vi "STM Read Message (Serial).vi"(6 "Options":T2={"Ignore Timeout Error"=TRUE, "timeout ms (1000)"=1000}, 8 "error in":errorcluster, 11 "Connection Info":T4) -> (0 "error out":errorcluster, 1 "Name":T3, 2 "data string":string, 3 "Connection Info Out":T4, 4 "Data Info":T1, 5 "Timed Out?":bool)   [LabVIEW 2014, in "QwaveSys Raspberry Pi Library.lvlib"]
doc: "This VI reads an incoming package of data from a host. This VI parses the package and extracts the data name and type as described in the meta data.\n\nFor the package to be parsed correctly, the meta data must be consistent in both the sender and the receiver. The data is packaged based on the existing meta data on the sender. \n\nUse the \"STM Read Meta Data\" and \"STM Write Meta Data\" VIs to ensure that both client and server have the same meta data.\n\nThe data is returned as a string. It is the responsibility of the user to cast it to the appropriate type."
uses:
  QwaveSys Raspberry Pi Library.lvlib
  stm_Serial Connection Info.ctl
  _SubVIs/stm_MetaDataElement.ctl
  stm_Serial Read Options.ctl
  stm_Serial Data Info.ctl
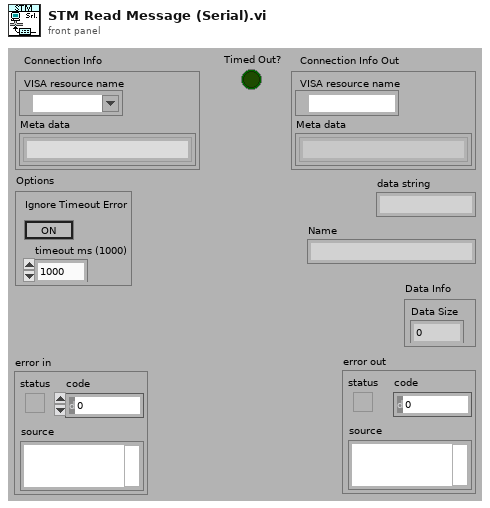
[diagram p1: front panel]
types:
  T1 = typedef "QwaveSys Raspberry Pi Library.lvlib/stm_Serial Data Info.ctl" = cluster{"Data Size":u32}
  T2 = typedef "QwaveSys Raspberry Pi Library.lvlib/stm_Serial Read Options.ctl" = cluster{"Ignore Timeout Error":bool, "timeout ms (1000)":u32}
  T3 = typedef "QwaveSys Raspberry Pi Library.lvlib/stm_MetaDataElement.ctl" = string
  T4 = typedef "QwaveSys Raspberry Pi Library.lvlib/stm_Serial Connection Info.ctl" = cluster{"VISA resource name":refnum<visa-resource-name>, "Meta data":T3[]}
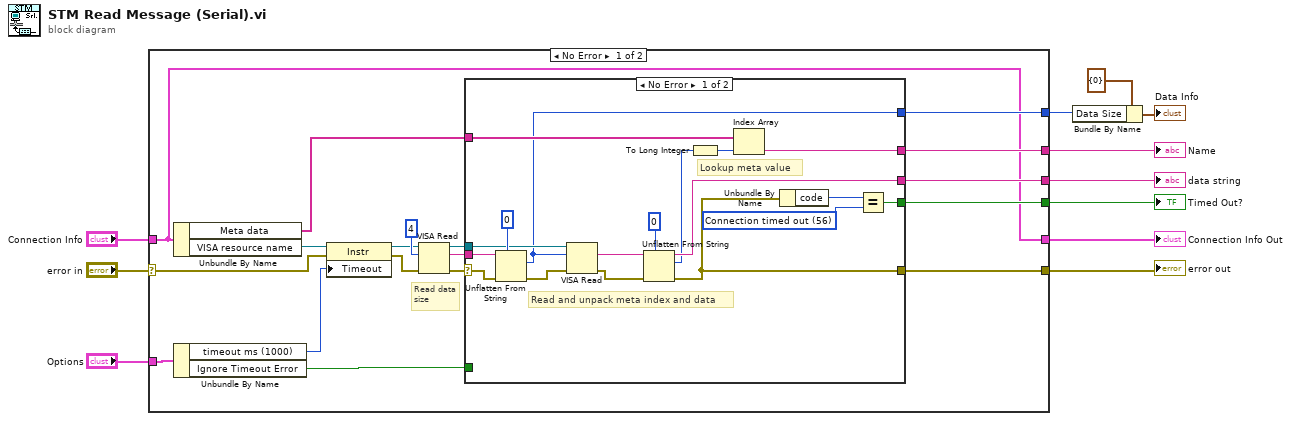
[diagram p0: block diagram]
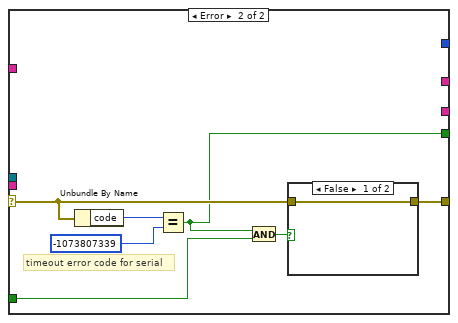
[diagram p2: hidden frame]
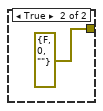
[diagram p3: hidden frame]
diagram:
  n1 = case shown="No Error" "error in" {
    selector: "error in" -> [w15 w57]
    tunnel: "Connection Info" -> [w12 w58]
    tunnel: [w12 w58] -> w11
    tunnel: [w25 w57] -> w10
    tunnel: [w24 _] -> w9
    tunnel: [w23 _] -> w8
    tunnel: [w22 _] -> w7
    tunnel: [w21 _] -> w3
    tunnel: "Options" -> [w18 _]
    frame No Error {
      # "Read data size"
      n2 = Unbundle By Name(w12) -> ("Meta data"=w19:T3[], "VISA resource name"=w17:refnum<visa-resource-name>)
      n3 = Unbundle By Name(w18) -> ("timeout ms (1000)"=w16:u32, "Ignore Timeout Error"=w20:bool)
      n4 = property class="Instr"(reference=w17, error in=w15, "Timeout"=w16) -> (reference out=w13:refnum<visa-resource-name>, error out=w14:errorcluster)
      n5 = VISA Read(VISA resource name=w13, byte count=u32 4 ("bytes to read"), error in (no error)=w14) -> (VISA resource name out=w27:refnum<visa-resource-name>, read buffer=w28:string, error out=w26:errorcluster)  [unwired: 1 out]
      n6 = case shown="No Error" w26 {
        selector: w26 -> [w40 w50]
        tunnel: w28 -> [w41 _]
        tunnel: w27 -> [w46 _]
        tunnel: w19 -> [w45 _]
        tunnel: [w38 w51] -> w25
        tunnel: w20 -> [_ w53]
        tunnel: [w42 w49] -> w24
        tunnel: [w37 _] -> w23
        tunnel: [w32 _] -> w22
        tunnel: [w36 _] -> w21
        frame No Error {
          w43 = 56 items=["No Error", "Argument Error", "Memory Full", "Out of Zone", "End of File", "File Already Open", "Generic File IO Error", "File Not Found", "File Permission Error", "Disk Full", "Duplicate Path", "Too Many Files Open", "Not Enabled", "Resource File Not Found", "Cannot Add Resource", "Resource Not Found", "Image Not Found", "Image Memory Error", "Pen Does Not Exist", "Config Bad Type", "Config Token Not Found", "Config Parse Error", "Config Memory Error", "Bad External Code Format", "Bad External Code Offset", "External Code Not Present", "Null Window", "Destroy Window Mixup", "Null Menu", "Print Aborted", "Bad Print Record", "Print Driver Error", "Windows Error During Print", "Memory Error During Print", "Print Dialog Error", "Generic Print Error", "Invalid Device Refnum", "Device Not Found", "Device Parameter Error", "Device Unit Error", "Can't Open Device", "Device Call Aborted", "Generic Error", "Cancelled By User", "Object ID Too Low", "Object ID Too High", "Object Not In Heap", "Unknown Heap", "Bad DefProc ID", "DefProc Not In Table", "Message Out Of Range", "Null Method", "Unknown Message", "Manager Call Not Supported", "Bad address", "Connection In progress", "Connection timed out", "Connection is already in progress", "Network attribute not supported", "Network error", "Address in use", "System out of memory", "Connection aborted", "Connection refused", "Connection is not connected", "Connection is already connected", "Connection closed", "Initialize error (interapplication manager)", "Bad occurrence", "Wait on unbound occurrence handler", "Occurrence queue overflow", "Bad path", "Semaphore not signaled", "Unrecognized type (interapplication manager)"] ("1st Error to Convert")
          # "Lookup meta value"
          # "Read and unpack meta index and data"
          n7 = Unflatten From String(type=u32 0 ("bytes to read"), binary string=w41, error in (no error)=w40) -> (value=w36:u32, error out=w34:errorcluster)  [unwired: 1 in, 2 out]
          n8 = VISA Read(VISA resource name=w46, byte count=w36, error in (no error)=w34) -> (read buffer=w35:string, error out=w39:errorcluster)  [unwired: 2 out]
          n9 = Unflatten From String(type=u16 0 ("bytes to read"), binary string=w35, error in (no error)=w39) -> (rest of the binary string=w32:string, value=w30:u16, error out=w38:errorcluster)  [unwired: 2 out]
          n10 = To Long Integer(number=w30) -> (32bit integer=w31:i32)
          n11 = Index Array(array=w45, index=w31) -> (element=w37:T3)
          n12 = Unbundle By Name(w38) -> ("code"=w44:i32)
          n13 = Equal?(x=w44, y=w43) -> (x = y?=w42:bool)
        }
        frame Error {
          # "timeout error code for serial"
          n14 = Unbundle By Name(w50) -> ("code"=w54:i32)
          n15 = Equal?(x=w54, y=-1073807339) -> (x = y?=w49:bool)
          n16 = And(x=w49, y=w53) -> (x .and. y?=w52:bool)
          n17 = case shown="False" w52 {
            tunnel: [w55 errorcluster {"status"=FALSE, "code"=0, "source"=""} ("error out")] -> w51
            tunnel: w50 -> [w55 _]
            frame False {
            }
            frame True {
            }
          }
        }
      }
    }
    frame Error {
    }
  }
  "error out" <- w10
  "Connection Info Out" <- w11
  "Timed Out?" <- w9
  "data string" <- w7
  "Name" <- w8
  n18 = Bundle By Name(cluster=T1 {"Data Size"=0} ("Data Info"), "Data Size"=w3) -> (→"Data Info":T1)
